vi "tcp_query_v2.vi"() -> ()   [LabVIEW 2019]
panel:
  out "status":bool
  out "EOS":bool=TRUE
  out "BOS":bool=TRUE
  out "client_step":i32
  in  "stop_query":bool
  out "spill_id":i32
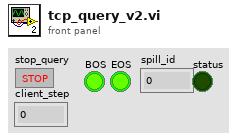
[diagram p1: front panel]
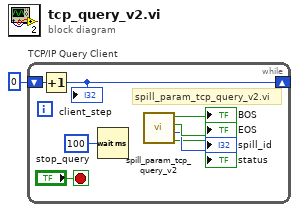
[diagram p0: block diagram]
diagram:
  n1 = while "TCP/IP Query Client" {
    shift-right: [w7] -> _
    shift-left: 0 -> [w8]
    stop <- "stop_query" stop-if-true
    # "spill_param_tcp_query_v2.vi"
    n2 = Increment(x=w8) -> (x+1=w7:i32)
    "client_step" <- w7
    n3 = Wait (ms)(milliseconds to wait=u32 100) -> ()  [unwired: 1 out]
    n4 = call "spill_param_tcp_query_v2.vi"() -> ("status"=→"status":bool, "spill_id"=→"spill_id":i32, "EOS"=→"EOS":bool, "BOS"=→"BOS":bool)  [unwired: 6 in]
  }
